vi "Autotrace Test.vi"() -> ()   [LabVIEW 2020]
uses:
  Autotrace Test Parameter.ctl
  Labview Library/Libraries/Basic Experiment/Basic Experiment.lvlib
panel:
  in  "Final\nWait":u32=5000
  in  "wait":u32=20
  in  "First\nWait":u32=3000
  out "Peak Position OneAxis AutoTrace":dbl(graph)
  out "Count Rate OneAxis AutoTrace":cluster{"Peak Count":dbl, "Final Count":dbl}(graph)
  in  "Stop Button":bool
  out "Stop Ref":refnum<vi>
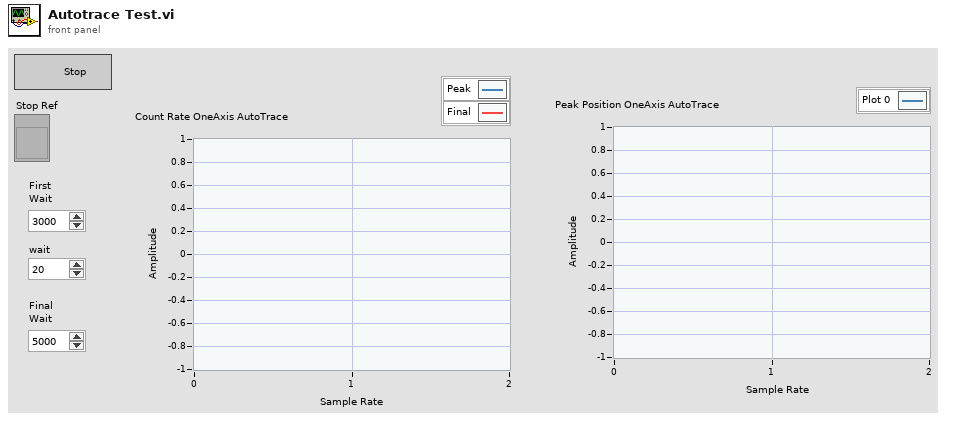
[diagram p1: front panel]
types:
  T1 = enum16{"Default", "Slow Mode", "User Config", "Test", "Run top", ""}
  T2 = typedef "Autotrace Test Parameter.ctl" = cluster{"Sample Rate (Hz)":dbl, "First\nWait":u32, "wait":u32, "Final\nWait":u32}
  T3 = enum32{"Bad", "Idle", "Run top level", "Running"}
  T4 = typedef "Basic Experiment.lvlib/1AutoTrace Results.ctl" = cluster{"Start Point":dbl, "Peak Position":dbl, "Final Count":dbl, "Peak Count":dbl, "Axis":enum16{"X", "Y", "Z"}, "Raw Tdms Path":path, "Raw Image Path":path, "Final Position":dbl, "Background":dbl}
  T5 = cluster{"Single AutoTrace Result":T4, "Background":dbl}
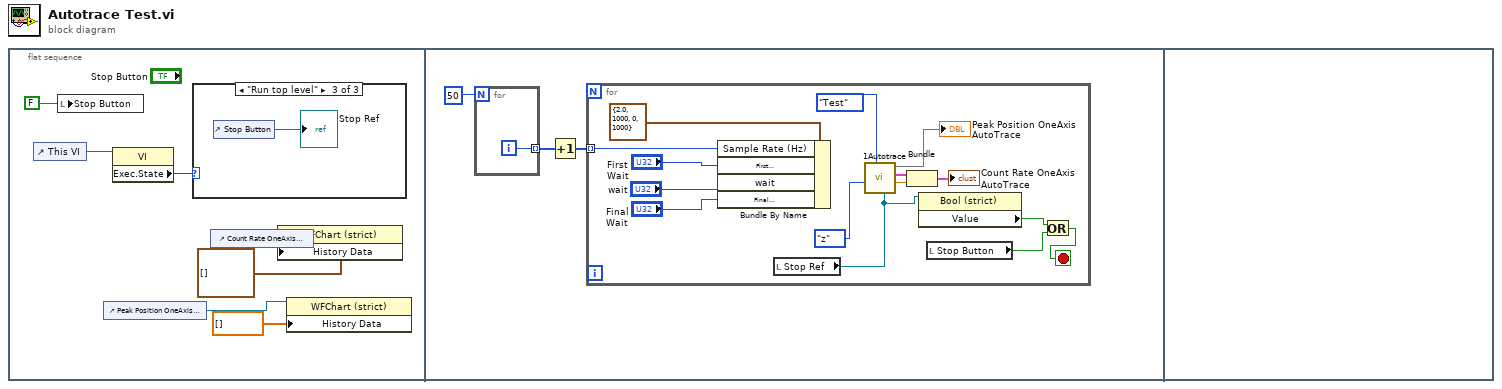
[diagram p0: block diagram]
diagram:
  n1 = flat-sequence {
    frame #0 {
      n2 = control-ref of="This VI"() -> (w5:refnum<vi>)
      n3 = local write "Stop Button"(FALSE) -> ()
      n4 = control-ref of="Peak Position OneAxis AutoTrace"() -> (w1:refnum<vi>)
      n5 = property class="VI"(reference=w5) -> ("Exec.State"=w6:T3)  [unwired: 1 in, 2 out]
      n6 = case shown="\"Run top level\"" w6 {
        frame "Bad", Default {
        }
        frame "Idle" {
        }
        frame "Run top level" {
          n7 = control-ref of="Stop Button"() -> (→"Stop Ref":refnum<vi>)
        }
      }
      n8 = control-ref of="Count Rate OneAxis AutoTrace"() -> (w4:refnum<vi>)
      n9 = property class="WFChart (strict)"(reference=w4, "History Data"=cluster{"Peak Count":dbl, "Final Count":dbl}[] []) -> ()  [unwired: 1 in, 2 out]
      n10 = property class="WFChart (strict)"(reference=w1, "History Data"=dbl[] []) -> ()  [unwired: 1 in, 2 out]
    }
    frame #1 {
      n11 = for {
        N: 50 -> [_]
        tunnel: [w12] -> w10 mode=indexing
        i -> [w12]
      }
      n12 = Increment(x=w10) -> (x+1=w9:i32[])
      n13 = for {
        tunnel: w9 -> [w23] mode=indexing
        stop <- w15 stop-if-true
        n14 = Bundle By Name(cluster=T2 {"Sample Rate (Hz)"=2.0, "First\nWait"=1000, "wait"=0, "Final\nWait"=1000} ("AutoTrace Test Parameter"), "Sample Rate (Hz)"=w23, "First\nWait"="First\nWait", "wait"="wait", "Final\nWait"="Final\nWait") -> ()  [unwired: 1 out]
        n15 = local read "Stop Ref"() -> (w18:refnum<vi>)
        n16 = call "1Autotrace.vi"(4:w18, "Mode"=T1."Test", 9:enum16{"x", "y", "z"}."z" ("Axis")) -> ("Background"=w20:dbl, "Single AutoTrace Result"=w21:T4, 3:→"Peak Position OneAxis AutoTrace")  [unwired: 5 in, 1 out]
        n17 = Bundle("Single AutoTrace Result"=w21, "Background"=w20) -> (→"Count Rate OneAxis AutoTrace":T5)  [unwired: 1 in]
        n18 = property class="Bool (strict)"(reference=w18) -> ("Value"=w17:bool)  [unwired: 1 in, 2 out]
        n19 = local read "Stop Button"() -> (w16:bool)
        n20 = Or(x=w17, y=w16) -> (x .or. y?=w15:bool)
      }
    }
    frame #2 {
    }
  }
